vi "Path1.vi"() -> ()   [LabVIEW 2018]
panel:
  out "路径文件夹":path
  in  "名称或相对路径":string
  out "输出的路径":path
  in  "路径":path
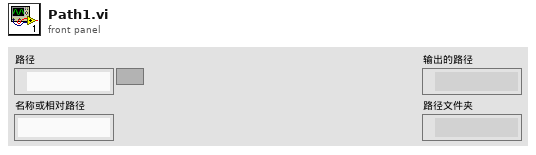
[diagram p1: front panel]
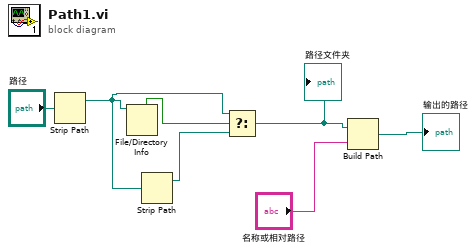
[diagram p0: block diagram]
diagram:
  n1 = Strip Path(path="路径") -> (stripped path=w5:path)  [unwired: 1 out]
  n2 = File/Directory Info(path=w5) -> (directory=w6:bool)  [unwired: 1 in, 6 out]
  n3 = Strip Path(path=w5) -> (stripped path=w4:path)  [unwired: 1 out]
  n4 = Select(t=w5, s=w6, f=w4) -> (s? t:f=w3:path)
  "路径文件夹" <- w3
  n5 = Build Path(base path=w3, name or relative path="名称或相对路径") -> (appended path=→"输出的路径":path)
